vi "Remove APU.vi"(8 "error in (no error)":errorcluster, 11 "APU Node":refnum<k24>) -> (0 "error out":errorcluster)   [LabVIEW 2015, in "Engine Simulation Toolkit SysDef API.lvlib"]
uses:
  Engine Simulation Toolkit SysDef API.lvlib
  NationalInstruments.VeriStand.SystemDefinitionAPI
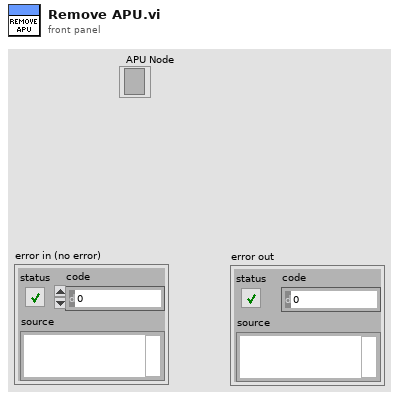
[diagram p1: front panel]
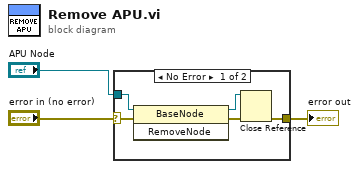
[diagram p0: block diagram]
diagram:
  n1 = case shown="No Error" "error in (no error)" {
    selector: "error in (no error)" -> [w8 w9]
    tunnel: [w5 w9] -> w3
    tunnel: "APU Node" -> [w7 _]
    frame No Error {
      n2 = invoke class="BaseNode" method="RemoveNode"(reference=w7, error in=w8) -> (reference out=w4:refnum<k24>, error out=w6:errorcluster)  [unwired: 1 in, 1 out]
      n3 = Close Reference(reference=w4, error in (no error)=w6) -> (error out=w5:errorcluster)
    }
    frame Error {
    }
  }
  "error out" <- w3
